vi "SubVI_Moving Ave.vi"(6 "Ave. NO":i32, 11 "Data":dbl[](array[numeric])) -> (3 "Filtered Data":dbl[](array[numeric]))   [LabVIEW 2013]
uses:
  <vilib>/Analysis/baseanly.llb/Mean (DBL).vi
  <vilib>/Analysis/NI_AALBase.lvlib
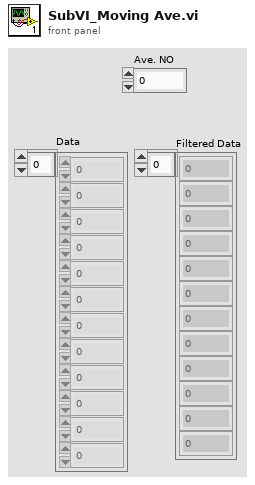
[diagram p1: front panel]
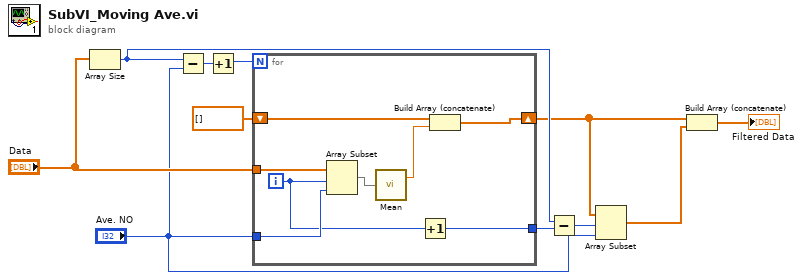
[diagram p0: block diagram]
diagram:
  n1 = Array Size(array="Data") -> (size(s)=w3:i32)
  n2 = Subtract(x=w3, y="Ave. NO") -> (x-y=w10:i32)
  n3 = Increment(x=w10) -> (x+1=w9:i32)
  n4 = for {
    N: w9 -> [_]
    tunnel: "Data" -> [w14]
    tunnel: "Ave. NO" -> [w19]
    shift-right: [w16] -> w1
    shift-left: dbl[] [] -> [w15]
    tunnel: [w12] -> w4
    i -> [w13]
    n5 = Array Subset(array=w14, index=w13, length=w19) -> (w18:dbl[])
    n6 = call-poly <vilib>:"Mean.vi"("X"=w18) -> ("mean"=w17:dbl)  [unwired: 1 out]
    n7 = Increment(x=w13) -> (x+1=w12:i32)
    n8 = Build Array (concatenate)(w15, w17) -> (w16:dbl[])
  }
  n9 = Subtract(x=w3, y=w4) -> (x-y=w2:i32)
  n10 = Array Subset(array=w1, index=w2, length="Ave. NO") -> (w5:dbl[])
  n11 = Build Array (concatenate)(w1, w5) -> (→"Filtered Data":dbl[])
